vi "Convert pixels to mm.vi"(2 "scale factor (mm / pixel)":dbl, 3 "camera angle, ccw+ rel. to trav. (deg)":dbl, 4 "dy (pix)":dbl, 5 "dx (pix)":dbl) -> (0 "dy (mm)":dbl, 1 "dx (mm)":dbl)   [LabVIEW 2014]
panel:
  # "Paul Nathan 11/06/2015"
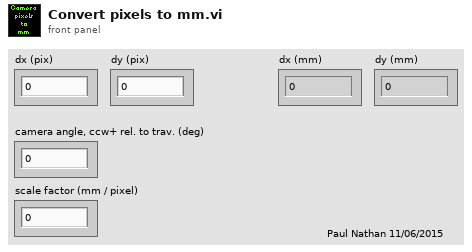
[diagram p1: front panel]
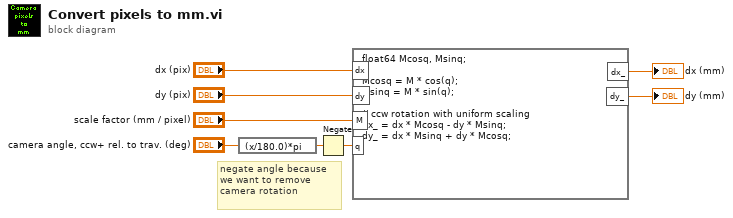
[diagram p0: block diagram]
diagram:
  # "negate angle because we want to remove camera rotation"
  n1 = expression code="(x/180.0)*pi" ("degrees to radians")("camera angle, ccw+ rel. to trav. (deg)") -> (w7:dbl)
  n2 = Negate(x=w7) -> (-x=w1:dbl)
  n3 = formula code="float64 Mcosq, Msinq;\n\nMcosq = M * cos(q);\nMsinq = M * sin(q);\n\n// ccw rotation with uniform scaling\ndx_ = dx * Mcosq - dy * Msinq;\ndy_ = dx * Msinq + dy * Mcosq;"("M"="scale factor (mm / pixel)", "q"=w1, "dy"="dy (pix)", "dx"="dx (pix)") -> ("dx_"=→"dx (mm)":dbl, "dy_"=→"dy (mm)":dbl)
